vi "getAll.vi"(8 "error in (no error)":errorcluster, 11 "Instrument.Oxford1820 in":refnum<class "Instrument.Oxford1820.lvclass">) -> (0 "error out":errorcluster, 2 "getAll":variant, 3 "Instrument.Oxford1820 out":refnum<class "Instrument.Oxford1820.lvclass">)   [LabVIEW 2016, in "Instrument.Oxford1820.lvclass"]
uses:
  Instrument.Oxford1820.lvclass
  Instrument.Oxford1820.lvclass/Instrument.Oxford1820.ctl
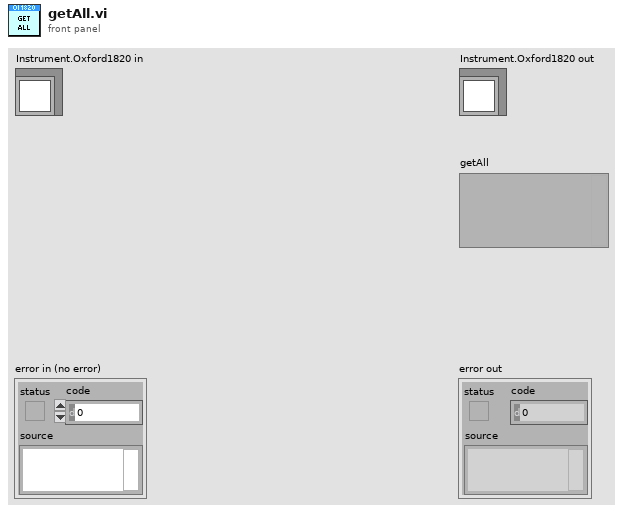
[diagram p1: front panel]
types:
  T1 = typedef "Instrument.Oxford1820.lvclass/getAll.ctl" = cluster{"1820_IPS_Magnet_Field":dbl, "1820_IPS_PS_Field":dbl, "1820_IPS_Target_Field":dbl, "1820_IPS_Target_Field_Rate":dbl, "1820_IPS_Voltage":dbl, "1820_IPS_Current":dbl, "1820_IPS_Level_N2":dbl, "1820_IPS_Level_He":dbl, "1820_IPS_Magnet_Temperature":dbl, "1820_IPS_Magnet_Temperature_R":dbl, "1820_IPS_M1_Current":dbl, "1820_IPS_M1_Voltage":dbl, "1820_IPS_M2_Current":dbl, "1820_IPS_M2_Voltage":dbl, "1820_IPS_M3_Current":dbl, "1820_IPS_M3_Voltage":dbl, "1820_IPS_Status":string, "1820_IPS_Switch":string, "1820_ITC_Lambda_Temperature":dbl, "1820_ITC_Lambda_Temperature_R":dbl, "1820_ITC_Pressure":dbl, "1820_ITC_Needle_Valve":dbl}
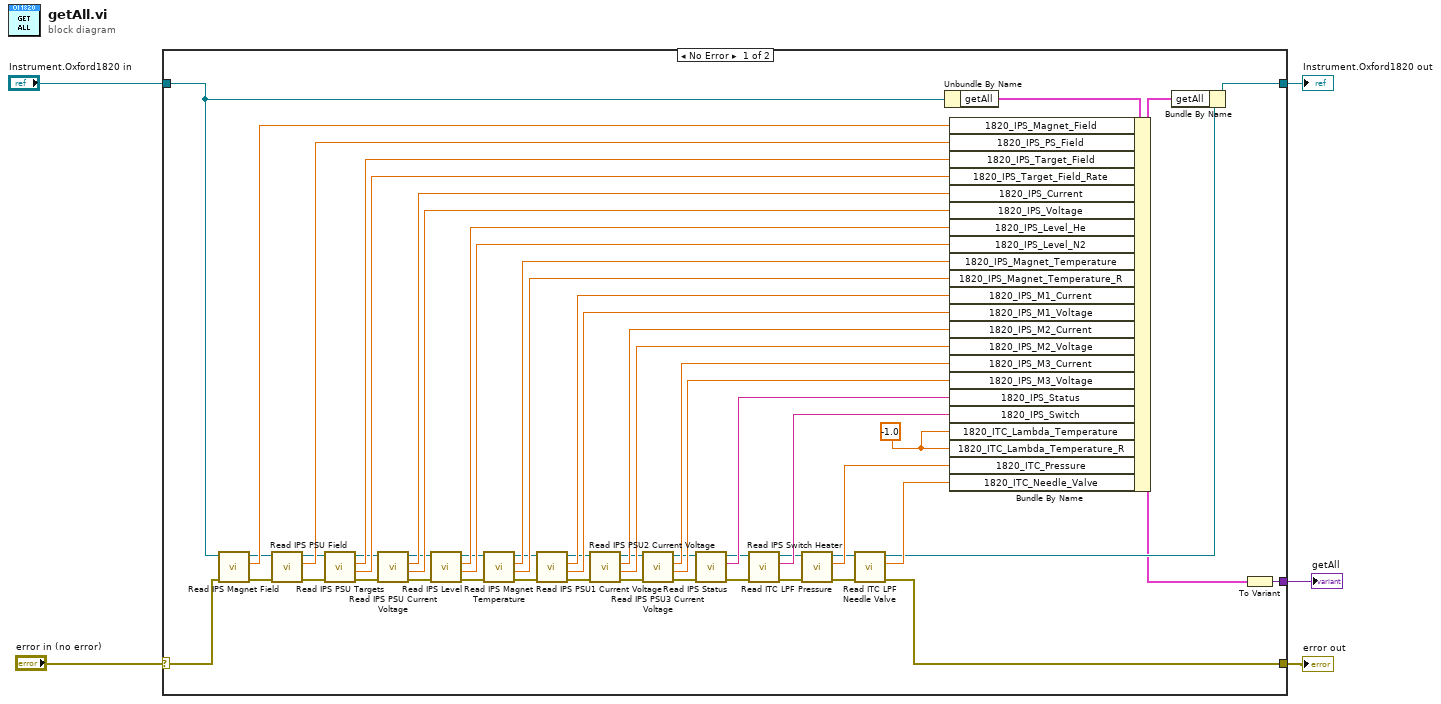
[diagram p0: block diagram]
diagram:
  n1 = case shown="No Error" "error in (no error)" {
    selector: "error in (no error)" -> [w37 w59]
    tunnel: "Instrument.Oxford1820 in" -> [w6 w60]
    tunnel: [w10 w60] -> w4
    tunnel: [w36 w59] -> w2
    tunnel: [w8 _] -> w1
    frame No Error {
      w57 = -1.0 ("getAll.1820_ITC_Lambda_Temperature")
      n2 = call "Read IPS Magnet Field.vi"("error in (no error)"=w37, "Instrument.Oxford1820 in"=w6) -> ("error out"=w34:errorcluster, "Magnet Field (T)"=w58:dbl, "Instrument.Oxford1820 out"=w35:refnum<class "Instrument.Oxford1820.lvclass">)  [unwired: 7 in]
      n3 = call "Read IPS PSU Field.vi"("error in (no error)"=w34, "Instrument.Oxford1820 in"=w35) -> ("error out"=w32:errorcluster, "Power Supply Field (T)"=w56:dbl, "Instrument.Oxford1820 out"=w33:refnum<class "Instrument.Oxford1820.lvclass">)  [unwired: 7 in]
      n4 = call "Read IPS PSU Targets.vi"("error in (no error)"=w32, "Instrument.Oxford1820 in"=w33) -> ("error out"=w30:errorcluster, "Target Field Rate (T/min)"=w54:dbl, "Target Field (T)"=w55:dbl, "Instrument.Oxford1820 out"=w31:refnum<class "Instrument.Oxford1820.lvclass">)  [unwired: 6 in]
      n5 = call "Read IPS PSU Current Voltage.vi"("error in (no error)"=w30, "Instrument.Oxford1820 in"=w31) -> ("error out"=w28:errorcluster, "Voltage (V)"=w52:dbl, "Current (A)"=w53:dbl, "Instrument.Oxford1820 out"=w29:refnum<class "Instrument.Oxford1820.lvclass">)  [unwired: 6 in]
      n6 = call "Read IPS Level.vi"("error in (no error)"=w28, "Instrument.Oxford1820 in"=w29) -> ("error out"=w26:errorcluster, "N2 Level (%)"=w50:dbl, "He Level (%)"=w51:dbl, "Instrument.Oxford1820 out"=w27:refnum<class "Instrument.Oxford1820.lvclass">)  [unwired: 6 in]
      n7 = call "Read IPS Magnet Temperature.vi"("error in (no error)"=w26, "Instrument.Oxford1820 in"=w27) -> ("error out"=w24:errorcluster, "Resistance (Ohms)"=w48:dbl, "Temperature (K)"=w49:dbl, "Instrument.Oxford1820 out"=w25:refnum<class "Instrument.Oxford1820.lvclass">)  [unwired: 6 in]
      n8 = call "Read IPS PSU1 Current Voltage.vi"("error in (no error)"=w24, "Instrument.Oxford1820 in"=w25) -> ("error out"=w22:errorcluster, "Voltage (V)"=w46:dbl, "Current (A)"=w47:dbl, "Instrument.Oxford1820 out"=w23:refnum<class "Instrument.Oxford1820.lvclass">)  [unwired: 6 in]
      n9 = call "Read IPS PSU2 Current Voltage.vi"("error in (no error)"=w22, "Instrument.Oxford1820 in"=w23) -> ("error out"=w20:errorcluster, "Voltage (V)"=w44:dbl, "Current (A)"=w45:dbl, "Instrument.Oxford1820 out"=w21:refnum<class "Instrument.Oxford1820.lvclass">)  [unwired: 6 in]
      n10 = call "Read IPS PSU3 Current Voltage.vi"("error in (no error)"=w20, "Instrument.Oxford1820 in"=w21) -> ("error out"=w18:errorcluster, "Voltage (V)"=w42:dbl, "Current (A)"=w43:dbl, "Instrument.Oxford1820 out"=w19:refnum<class "Instrument.Oxford1820.lvclass">)  [unwired: 6 in]
      n11 = call "Read IPS Status.vi"("error in (no error)"=w18, "Instrument.Oxford1820 in"=w19) -> ("error out"=w16:errorcluster, "Status"=w41:string, "Instrument.Oxford1820 out"=w17:refnum<class "Instrument.Oxford1820.lvclass">)  [unwired: 7 in]
      n12 = call "Read IPS Switch Heater.vi"("error in (no error)"=w16, "Instrument.Oxford1820 in"=w17) -> ("error out"=w14:errorcluster, "Switch Heater Status"=w40:string, "Instrument.Oxford1820 out"=w15:refnum<class "Instrument.Oxford1820.lvclass">)  [unwired: 6 in, 1 out]
      n13 = call "Read ITC LPF Pressure.vi"("error in (no error)"=w14, "Instrument.Oxford1820 in"=w15) -> ("error out"=w12:errorcluster, "LPF Pressure (mbar)"=w39:dbl, "Instrument.Oxford1820 out"=w13:refnum<class "Instrument.Oxford1820.lvclass">)  [unwired: 7 in]
      n14 = call "Read ITC LPF Needle Valve.vi"("error in (no error)"=w12, "Instrument.Oxford1820 in"=w13) -> ("error out"=w36:errorcluster, "LPF Needle Valve (%)"=w38:dbl, "Instrument.Oxford1820 out"=w9:refnum<class "Instrument.Oxford1820.lvclass">)  [unwired: 7 in]
      n15 = Unbundle By Name(w6) -> ("getAll"=w11:T1)
      n16 = Bundle By Name(cluster=w11, "1820_IPS_Magnet_Field"=w58, "1820_IPS_PS_Field"=w56, "1820_IPS_Target_Field"=w55, "1820_IPS_Target_Field_Rate"=w54, "1820_IPS_Current"=w53, "1820_IPS_Voltage"=w52, "1820_IPS_Level_He"=w51, "1820_IPS_Level_N2"=w50, "1820_IPS_Magnet_Temperature"=w49, "1820_IPS_Magnet_Temperature_R"=w48, "1820_IPS_M1_Current"=w47, "1820_IPS_M1_Voltage"=w46, "1820_IPS_M2_Current"=w45, "1820_IPS_M2_Voltage"=w44, "1820_IPS_M3_Current"=w43, "1820_IPS_M3_Voltage"=w42, "1820_IPS_Status"=w41, "1820_IPS_Switch"=w40, "1820_ITC_Lambda_Temperature"=w57, "1820_ITC_Lambda_Temperature_R"=w57, "1820_ITC_Pressure"=w39, "1820_ITC_Needle_Valve"=w38) -> (w7:T1)
      n17 = Bundle By Name(cluster=w9, "getAll"=w7) -> (w10:refnum<class "Instrument.Oxford1820.lvclass">)
      n18 = To Variant(anything=w7) -> (Variant=w8:variant)
    }
    frame Error {
    }
  }
  "error out" <- w2
  "Instrument.Oxford1820 out" <- w4
  "getAll" <- w1
